vi "GetXMLImageServer.vi"(8 "error in":errorcluster, 11 "Node":refnum<k20>) -> (0 "error out":errorcluster, 3 "ImageServer":cluster{"IPAddress":string, "Port":i32})   [LabVIEW 2013]
uses:
  <vilib>/xml/NI_XML.lvlib
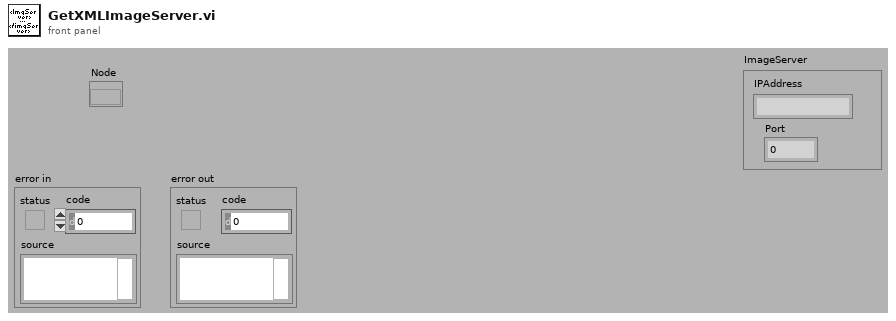
[diagram p1: front panel]
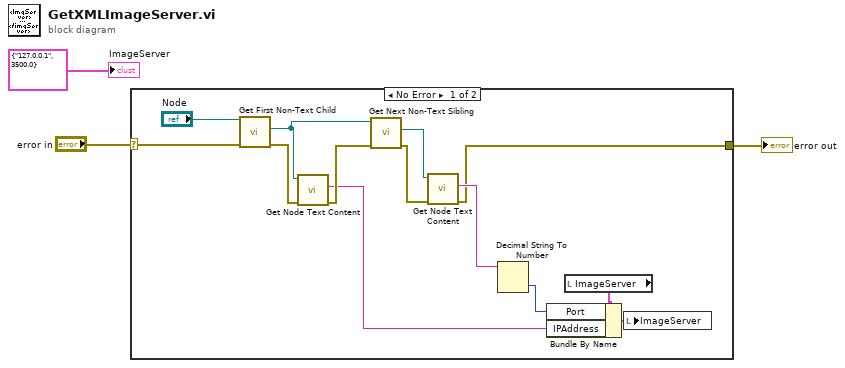
[diagram p0: block diagram]
diagram:
  n1 = case shown="No Error" "error in" {
    selector: "error in" -> [w10 w17]
    tunnel: [w6 w17] -> w2
    frame No Error {
      n2 = call <vilib>:"Get First Non-Text Child.vi"("error in (no error)"=w10, "node in"="Node") -> ("error out"=w15:errorcluster, "child node"=w4:refnum<k20>)  [unwired: 6 in, 2 out]
      n3 = call <vilib>:"Get Node Text Content.vi"("error in (no error)"=w15, "node in"=w4) -> ("error out"=w13:errorcluster, "node text"=w9:string)  [unwired: 7 in, 1 out]
      n4 = call <vilib>:"Get Next Non-Text Sibling.vi"("error in (no error)"=w13, "node in"=w4) -> ("error out"=w14:errorcluster, "sibling node"=w5:refnum<k20>)  [unwired: 6 in, 2 out]
      n5 = call <vilib>:"Get Node Text Content.vi"("error in (no error)"=w14, "node in"=w5) -> ("error out"=w6:errorcluster, "node text"=w8:string)  [unwired: 7 in, 1 out]
      n6 = Decimal String To Number(string=w8) -> (number=w7:i32)  [unwired: 2 in, 1 out]
      n7 = local read "ImageServer"() -> (w12:cluster{"IPAddress":string, "Port":i32})
      n8 = Bundle By Name(cluster=w12, "Port"=w7, "IPAddress"=w9) -> (w11:cluster{"IPAddress":string, "Port":i32})
      n9 = local write "ImageServer"(w11) -> ()
    }
    frame Error {
    }
  }
  "error out" <- w2
  "ImageServer" <- cluster{"IPAddress":string, "Port":dbl} {"IPAddress"="127.0.0.1", "Port"=3500.0} ("ImageServer")
